vi "Off.vi"(8 "error in (no error)":errorcluster, 11 "reference in":refnum<class "Light.lvclass">) -> (0 "error out":errorcluster, 3 "reference out":refnum<class "Light.lvclass">)   [LabVIEW 2020, in "Light.lvclass"]
uses:
  Light.lvclass
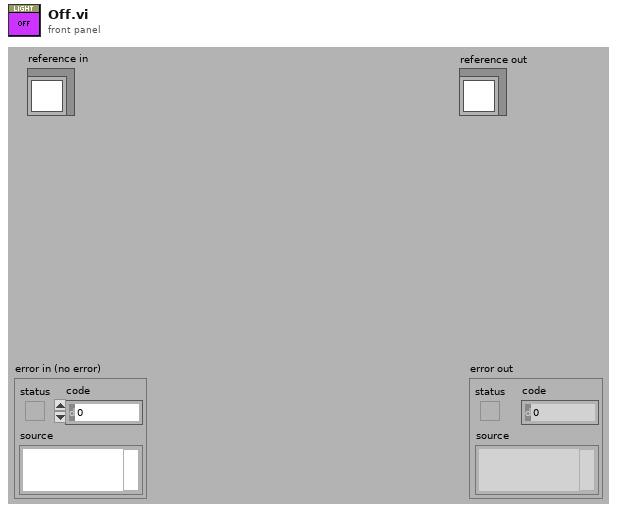
[diagram p1: front panel]
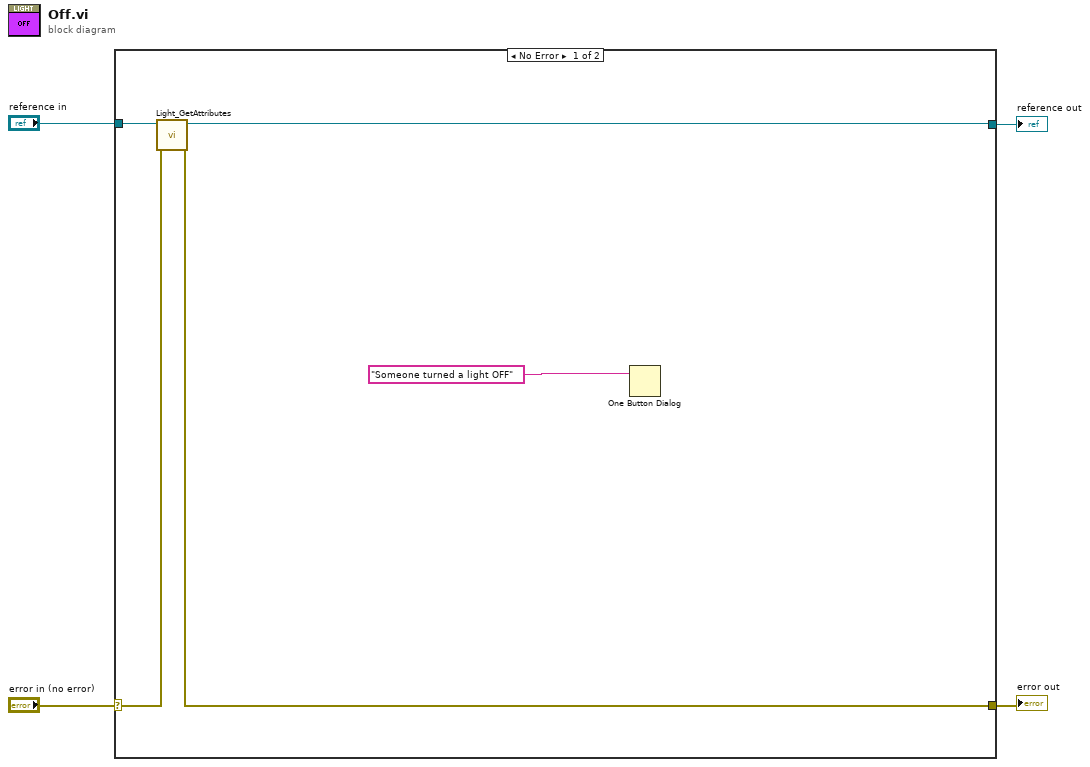
[diagram p0: block diagram]
diagram:
  n1 = case shown="No Error" "error in (no error)" {
    selector: "error in (no error)" -> [w8 w11]
    tunnel: [w6 w11] -> w3
    tunnel: [w7 w10] -> w1
    tunnel: "reference in" -> [w9 w10]
    frame No Error {
      n2 = call "Light_GetAttributes.vi"("error in (no error)"=w8, "reference in"=w9) -> ("error out"=w6:errorcluster, "reference out"=w7:refnum<class "Light.lvclass">)  [unwired: 6 in, 2 out]
      n3 = One Button Dialog(message="Someone turned a light OFF" ("TextIn")) -> ()  [unwired: 1 in, 1 out]
    }
    frame Error {
    }
  }
  "error out" <- w3
  "reference out" <- w1
